vi "main ui.vi"() -> ()   [LabVIEW 2015]
uses:
  type def/basic params.ctl
  type def/advanced params.ctl
  type def/imaging mode.ctl
  type def/PXI control.ctl
  <instrlib>/niScope/Controls/niScope trigger source digital.ctl
  type def/NI tasks.ctl
  type def/do waveform.ctl
  type def/task plan.ctl
  type def/task status.ctl
  type def/motor panel.ctl
  type def/stage plan.ctl
  C:/Users/Administrator/Desktop/labview program/sub vi/XPS-UNIFIED/LabVIEW VIs/LabVIEW Source Code/Dll/Newport.XPS.CommandInterface.dll
  sub vi/XPS-UNIFIED/LabVIEW VIs/LabVIEW Source Code/Dll/Newport.XPS.CommandInterface.dll
  global variables/params.vi
  <instrlib>/niScope/Acquire/Fetch/niScope Multi Fetch Binary 16.vi
panel:
  in  "bi? for display":bool=TRUE
  in  "bi? for save":bool=TRUE
  out "t":dbl
  out "speed":dbl
  out "Y end":dbl
  out "main trigger":refnum<k21>
  out "XPS Ref":refnum<k24>
  out "PMT2 array size":i32[](array[numeric])
  out "PMT array size":i32[](array[numeric])
  in  "Stop stage":bool=TRUE
  out "stage state":string="exit"
  in  "stage plan":T1[][](array[typedef])
  in  "motor panel":T2={"X neg"=FALSE, "X pos"=FALSE, "dZ"=0.01, "X destination"=0.0, "Y destination"=0.0, "Z destination"=0.0, "Y pos"=FALSE, "Y neg"=FALSE, "Blank"=FALSE, "Blank 2"=FALSE, "X"=0.0, "Y"=0.0, "Z"=0.0, "X go"=FALSE, "Y go"=FALSE, "Z go"=FALSE, "Z pos"=FALSE, "Z neg"=FALSE, "dXY"=0.5} {"dXY" min=0.0 max=3.0 step=0.0001 format="%#.4f"; "Z" format="%#_6f"; "Y" format="%#_6f"; "X" format="%#_6f"; "Z destination" min=-13.0 max=10.0 step=0.001 format="%.3f"; "Y destination" min=-25.0 max=25.0 step=0.001 format="%.3f"; "X destination" min=-25.0 max=25.0 step=0.001 format="%.3f"; "dZ" min=0.0 max=1.0 step=0.0001 format="%#.4f"}
  out "do waveforms":T3[](array[typedef])
  out "images":i16[][][](array[numeric])
  out "NI tasks":T4
  in  "imaging mode":T5="continuous imaging"
  out "file path":path
  out "current state":string="exit"
  in  "Calc Waveform":bool
  in  "Stop":bool=TRUE
  in  "Acquire":bool
  in  "tab param":enum32{"basic", "advanced", "PXI", "task "}(tab)
  in  "basic params":T6={"X pixel #"=200, "X pixel size(um)"=1.0, "Y pixel #"=200, "Y pixel size(um)"=10.0, "line rate(Hz)"=1.0, "stage scan?"=FALSE} {"line rate(Hz)" min=1.0 max=2000.0 format="%#.3g"; "X pixel size(um)" min=0.0 max=10.0 format="%#.3g"; "X pixel #" min=2 max=20480 step=2 format="%#.3g"; "Y pixel size(um)" min=0.0 max=10.0 format="%#.3g"; "Y pixel #" min=2 max=204800 step=2 format="%#.3g"}
  in  "advanced params":T7={"x flyback time(%)"=40.0, "signal offset"=0, "frame time(s)"=0.0, "fetch # per frame"=1, "galvo sampling rate"=500000} {"galvo sampling rate" min=10000 max=200000 step=1; "fetch # per frame" min=1 max=1000 step=1 format="%#.3g"; "frame time(s)" min=0.0 max=100.0 step=0.1 format="%#.3g"; "signal offset" max=10000 format="%#.3g"; "x flyback time(%)" min=0.0 max=50.0 format="%#.3g"}
  in  "PXI channel":T8={"Vertical Range (V)"=1.0, "Min Sample Rate"=2208791.906743315, "# of Channels"=1, "Min Record Length"=560, "Number Of Records"=10000, "Trigger Position(%)"=0.0, "act Record Length"=1000, "trigger source"="VAL_EXTERNAL", "PMT2 # of Channels"=1} {"PMT2 # of Channels" min=1 max=8 step=1; "act Record Length" min=0 max=100000 step=1 format="%#.3g"; "Trigger Position(%)" min=0.0 max=100.0 format="%#.3p"; "Number Of Records" min=0 max=1000000 step=1 format="%#.3g"; "Min Record Length" min=0 max=10000 step=1; "# of Channels" min=1 max=8 step=1; "Min Sample Rate" min=0.0 max=100000000.0 format="%#.3p"; "Vertical Range (V)" min=0.0 max=10.0 format="%#.3g"}
  in  "task plan":T10={"X start"=0.0, "X end"=0.0, "X overlap"=0.0, "Y start"=20.0, "Y end"=0.0, "Z start"=0.0, "Z end"=0.0, "Z step size"=0.0, "start scan #"=0, "end scan #"=0} {"end scan #" min=1 step=1; "start scan #" min=1 step=1; "Z step size" min=-10.0 max=10.0 format="%#.6g"; "Z end" min=-12.0 max=12.0; "Z start" min=-12.0 max=12.0; "Y end" min=-20.0 max=20.0; "Y start" min=-20.0 max=20.0; "X overlap" min=0.0; "X end" min=-20.0 max=20.0; "X start" min=-20.0 max=20.0}
  in  "test plan":bool
  in  "save plan":bool
  in  "load plan":bool
  out "task status":T11
  in  "tab image":enum32{"Image", "Waveform"}(tab)
  in  "PMT channel":u8
  out "image":T12(plugin-control)
  out "current frame index":u16 caption="cn" format="%#.3g"
  in  "max":i32 format="%#.3g"
  in  "min":i32 format="%#.3g"
  in  "convesion":u32(ring)=15 items=["90% Dynamic"=15, "Given Range"=14]
  in  "acquisition finished":bool
  out "Enable error":i32
  out "waveform":dbl[](graph)
  in  "channel":cluster{"channel #":dbl, "signal":string}
  # "X"
  # "Y"
  # "Z"
  # "write"
  # "scan"
  # "in"
  # "z block"
  # "in"
  # "x block"
  # "in"
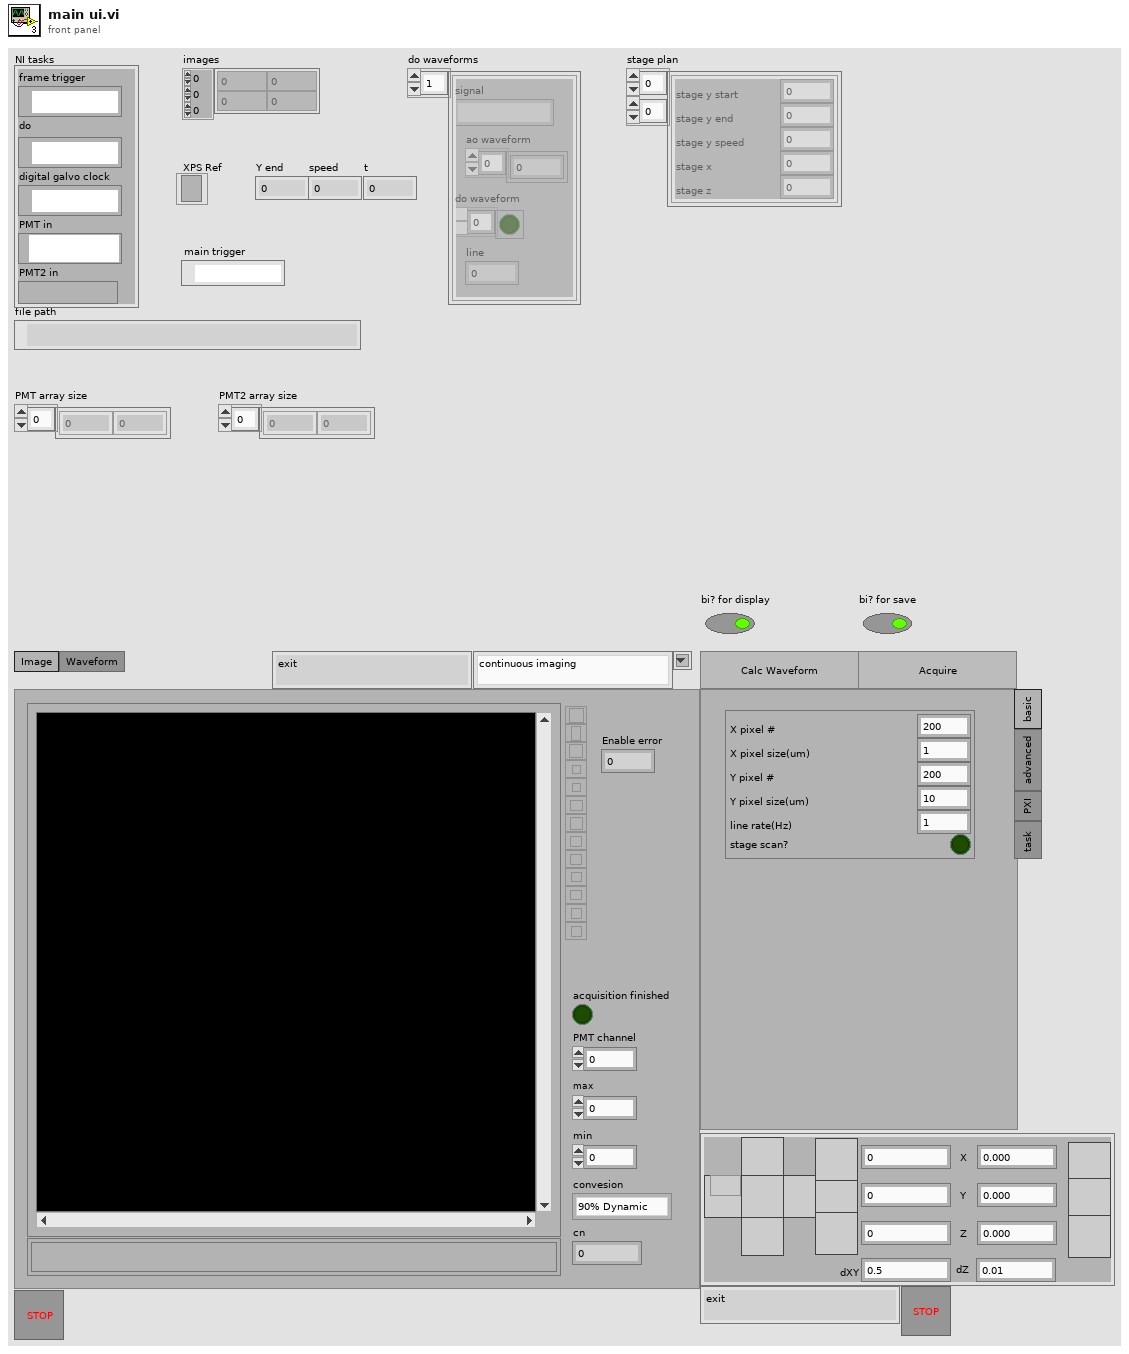
[diagram p1: front panel]
types:
  T1 = typedef "stage plan.ctl" = cluster{"stage y start":dbl, "stage y end":dbl, "stage y speed":dbl, "stage x":dbl, "stage z":dbl}
  T2 = typedef "motor panel.ctl" = cluster{"X neg":bool, "X pos":bool, "dZ":dbl, "X destination":dbl, "Y destination":dbl, "Z destination":dbl, "Y pos":bool, "Y neg":bool, "Blank":bool, "Blank 2":bool, "X":dbl, "Y":dbl, "Z":dbl, "X go":bool, "Y go":bool, "Z go":bool, "Z pos":bool, "Z neg":bool, "dXY":dbl}
  T3 = typedef "do waveform.ctl" = cluster{"signal":string, "ao waveform":dbl[], "do waveform":bool[], "line":u8}
  T4 = typedef "NI tasks.ctl" = cluster{"frame trigger":refnum<k21>, "do":refnum<k21>, "digital galvo clock":refnum<k21>, "PMT in":refnum<k15>, "PMT2 in":refnum<k15>}
  T5 = typedef "imaging mode.ctl" = string
  T6 = typedef "basic params.ctl" = cluster{"X pixel #":u32, "X pixel size(um)":dbl, "Y pixel #":u32, "Y pixel size(um)":dbl, "line rate(Hz)":dbl, "stage scan?":bool}
  T7 = typedef "advanced params.ctl" = cluster{"x flyback time(%)":dbl, "signal offset":u16, "frame time(s)":dbl, "fetch # per frame":u16, "galvo sampling rate":u32}
  T8 = typedef "PXI control.ctl" = cluster{"Vertical Range (V)":dbl, "Min Sample Rate":dbl, "# of Channels":u8, "Min Record Length":i32, "Number Of Records":i32, "Trigger Position(%)":dbl, "act Record Length":i32, "trigger source":T9, "PMT2 # of Channels":u8}
  T9 = typedef "niScope trigger source digital.ctl" = string
  T10 = typedef "task plan.ctl" = cluster{"X start":dbl, "X end":dbl, "X overlap":dbl, "Y start":dbl, "Y end":dbl, "Z start":dbl, "Z end":dbl, "Z step size":dbl, "start scan #":u16, "end scan #":u16}
  T11 = typedef "task status.ctl" = cluster{"xn":u16, "x total":u16, "zn":u16, "z total":u16, "scan n":u16, "scan total":u16, "write":u16}
  T12 = typedef "IMAQ Image.ctl" = refnum<image>
  T13 = enum8{"Enabled", "Disabled", "Disabled and Grayed Out"}
  T14 = typedef "Image Type" = u32
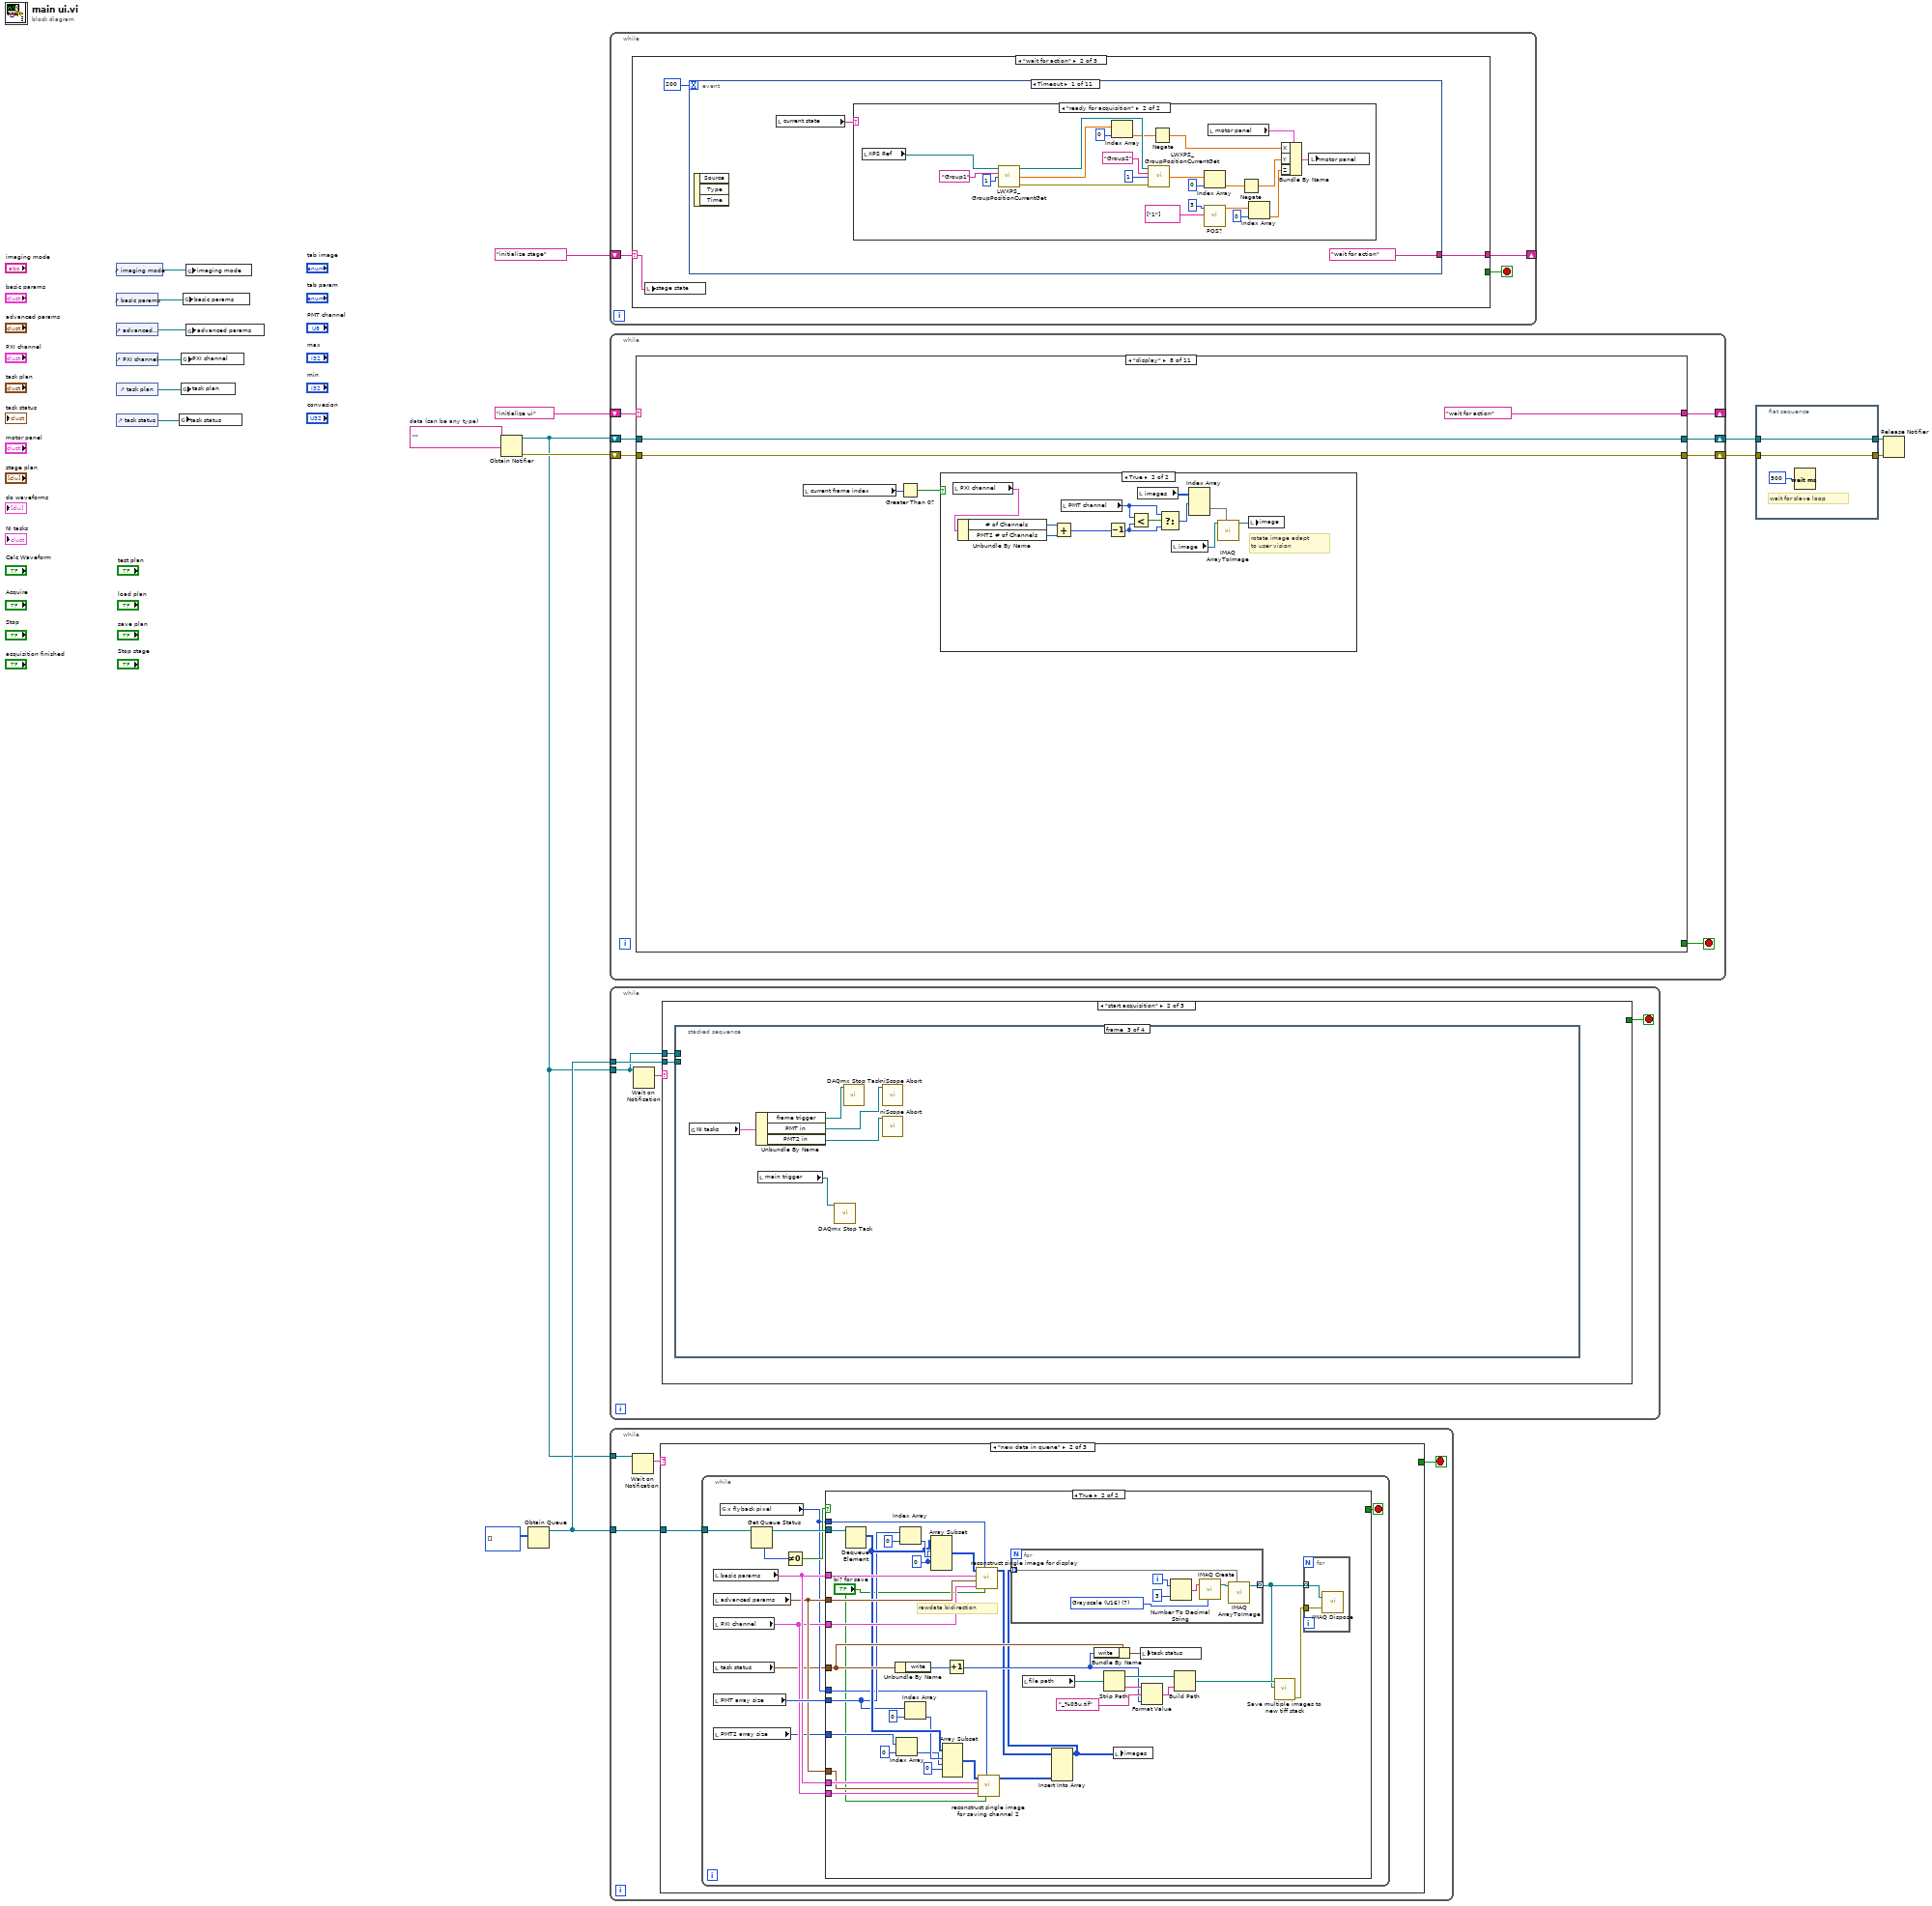
[diagram p0: block diagram]
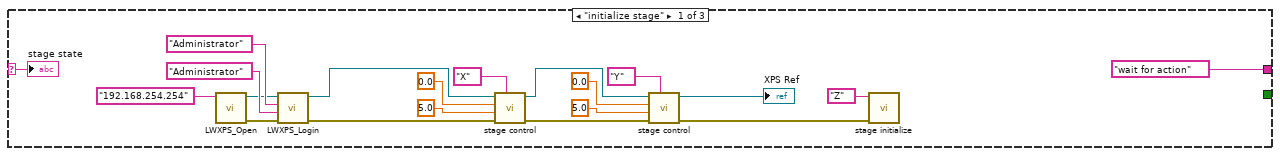
[diagram p2: hidden frame]
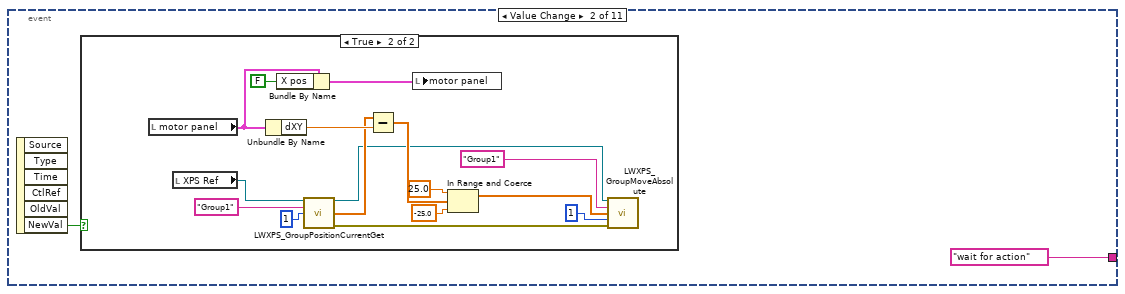
[diagram p4: hidden frame]
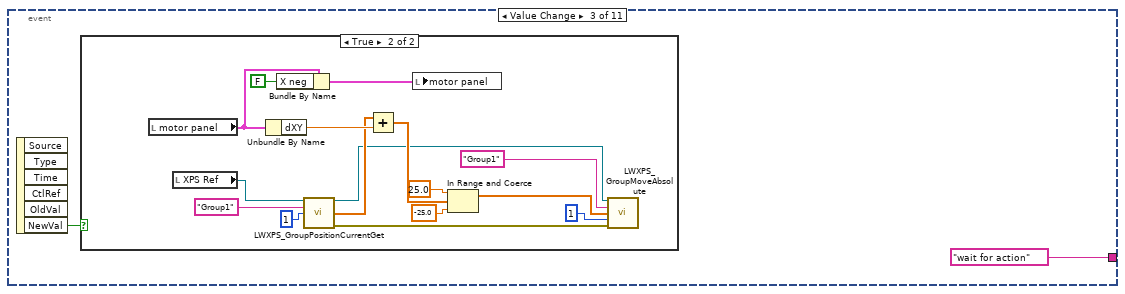
[diagram p6: hidden frame]
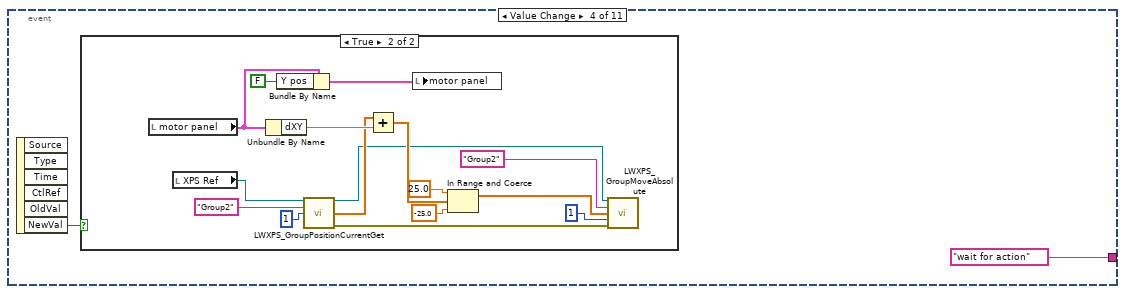
[diagram p8: hidden frame]
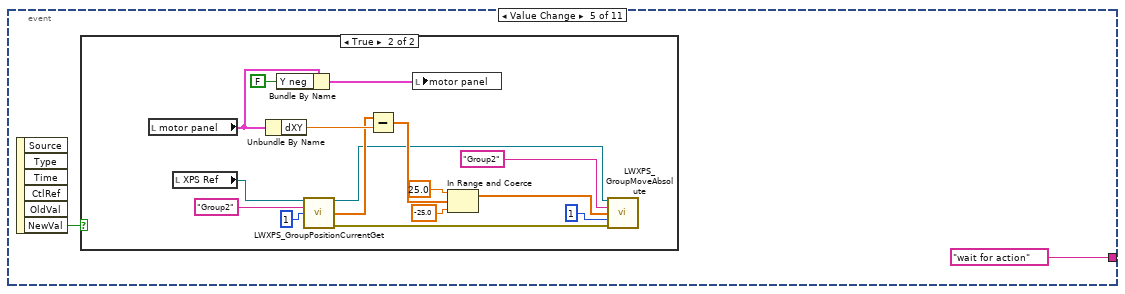
[diagram p10: hidden frame]
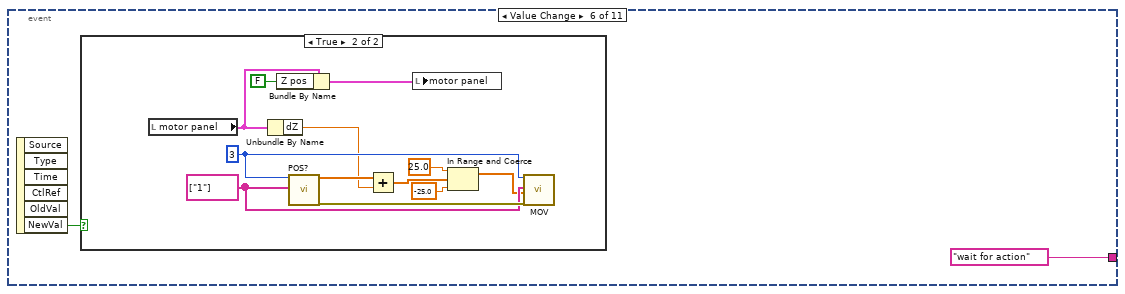
[diagram p12: hidden frame]
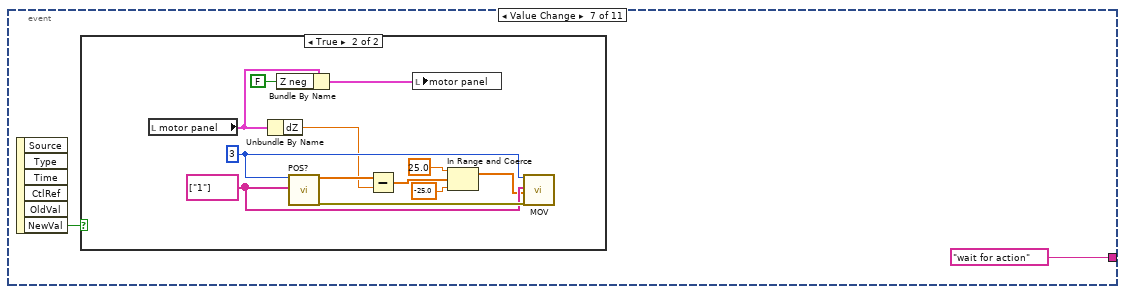
[diagram p14: hidden frame]
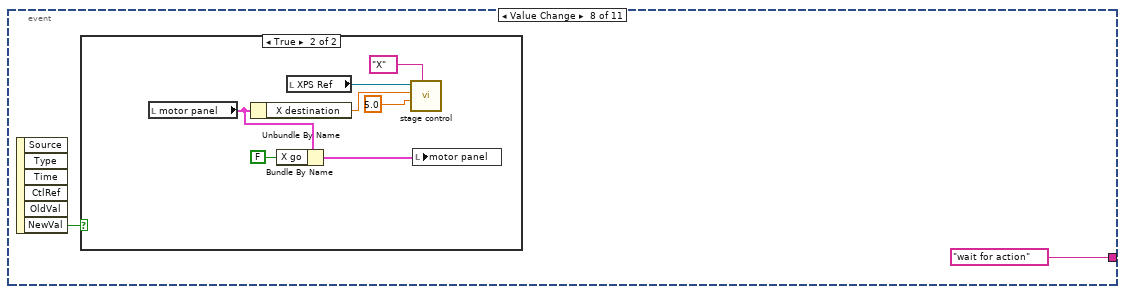
[diagram p16: hidden frame]
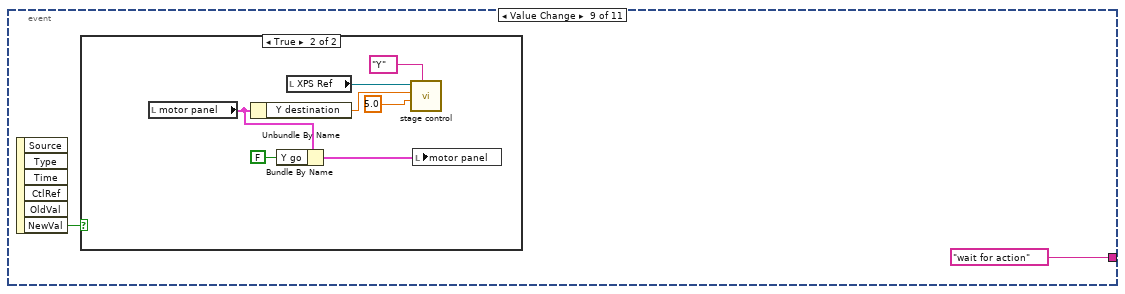
[diagram p18: hidden frame]
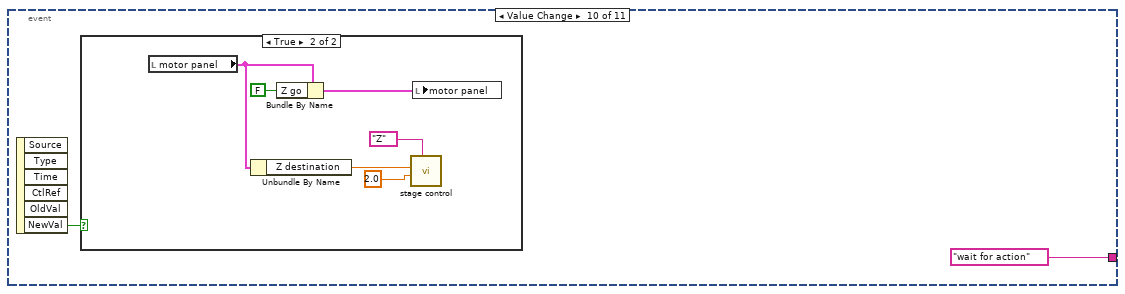
[diagram p20: hidden frame]
diagram:
  w16 = ""  # data (can be any type)
  n1 = control-ref of="imaging mode"() -> (w12:refnum<vi>)
  n2 = control-ref of="basic params"() -> (w14:refnum<vi>)
  n3 = control-ref of="advanced params"() -> (w13:refnum<vi>)
  n4 = control-ref of="PXI channel"() -> (w11:refnum<vi>)
  n5 = control-ref of="task plan"() -> (w4:refnum<vi>)
  n6 = control-ref of="task status"() -> (w2:refnum<vi>)
  n7 = global write "params.vi" "task status"(w2) -> ()
  n8 = global write "params.vi" "task plan"(w4) -> ()
  n9 = global write "params.vi" "PXI channel"(w11) -> ()
  n10 = global write "params.vi" "basic params"(w14) -> ()
  n11 = global write "params.vi" "imaging mode"(w12) -> ()
  n12 = global write "params.vi" "advanced params"(w13) -> ()
  n13 = Obtain Notifier(notification data type=w16) -> (notifier out=w3:refnum<notifier>, error out=w17:errorcluster)  [unwired: 2 in, 2 out]
  n14 = Obtain Queue(element data type=i16[][] []) -> (queue out=w10:refnum<queue>)  [unwired: 4 in, 2 out]
  n15 = while {
    shift-right: [w19] -> _
    shift-left: "initialize stage" -> [w20]
    stop <- w18 stop-if-true
    n16 = case shown="\"wait for action\"" w20 {
      selector: w20 -> [w40 w41 w200]
      tunnel: ["wait for action" w42 "exit"] -> w19
      tunnel: [_ _ TRUE] -> w18
      frame "initialize stage" {
        n17 = call "LWXPS_Open.vi"("Instrument Key IN"="192.168.254.254" ("address")) -> ("LabVIEW error OUT"=w35:errorcluster, "XPS Reference OUT"=w34:refnum<k24>)  [unwired: 3 in, 2 out]
        n18 = call "LWXPS_Login.vi"("LabVIEW error IN"=w35, "Password"="Administrator" ("User Name"), "User Name"="Administrator", "CommandInterfaceXPS.XPS"=w34) -> ("LabVIEW error OUT"=w32:errorcluster, "CommandInterfaceXPS.XPS"=w22:refnum<k24>)  [unwired: 2 in, 2 out]
        n19 = call "stage control.vi"("Combo Box"="X", "error in"=w32, "speed"=5.0, "target"=0.0, "XPS Ref in"=w22) -> ("error out"=w31:errorcluster, "XPS ref out"=w21:refnum<k24>)  [unwired: 5 in]
        n20 = call "stage control.vi"("Combo Box"="Y", "error in"=w31, "speed"=5.0, "target"=0.0, "XPS Ref in"=w21) -> ("error out"=w23:errorcluster, "XPS ref out"=→"XPS Ref":refnum<k24>)  [unwired: 5 in]
        n21 = call "stage initialize.vi"("error in"=w23, "Combo Box"="Z") -> ()  [unwired: 9 in, 1 out]
        "stage state" <- w40
      }
      frame "wait for action" {
        n22 = local write "stage state"(w41) -> ()
        n23 = event shown="[0] Timeout" {
          selector: _ -> [_ _ _ _ _ _ _ _ _ _ _]
          dyn-events: _ -> [_ _ _ _ _ _ _ _ _ _ _]
          timeout: 200 -> [_ _ _ _ _ _ _ _ _ _ _]
          tunnel: ["wait for action" "wait for action" "wait for action" "wait for action" "wait for action" "wait for action" "wait for action" "wait for action" "wait for action" "wait for action" "exit"] -> w42
          event Timeout {
            n24 = event-data() -> ()  [unwired: 1 in, 3 out]
            n25 = local read "current state"() -> (w44:string)
            n26 = case shown="\"ready for acquisition\"" w44 {
              frame "False", Default {
              }
              frame "ready for acquisition" {
                n27 = local read "XPS Ref"() -> (w47:refnum<k24>)
                n28 = call "LWXPS_GroupPositionCurrentGet.vi"("CommandInterfaceXPS.XPS"=w47, "Group Name"="Group1", "Number of positioners"=1) -> ("CommandInterfaceXPS.XPS"=w52:refnum<k24>, "Current Encoder Position"=w60:dbl[], "LabVIEW error OUT"=w46:errorcluster)  [unwired: 8 in, 2 out]
                n29 = Index Array(array=w60, index=0) -> (element=w51:dbl)
                n30 = call "LWXPS_GroupPositionCurrentGet.vi"("CommandInterfaceXPS.XPS"=w52, "Group Name"="Group2", "Number of positioners"=1, "LabVIEW error IN"=w46) -> ("Current Encoder Position"=w53:dbl[])  [unwired: 7 in, 4 out]
                n31 = Negate(x=w51) -> (-x=w50:dbl)
                n32 = Index Array(array=w53, index=0) -> (element=w48:dbl)
                n33 = call "POS?.vi"("System no."=3, "Axes to query"=string[] ["1"]) -> ("Position"=w59:dbl[])  [unwired: 3 in, 14 out]
                n34 = local read "motor panel"() -> (w67:T2)
                n35 = Negate(x=w48) -> (-x=w49:dbl)
                n36 = Index Array(array=w59, index=0) -> (element=w66:dbl)
                n37 = Bundle By Name(cluster=w67, "X"=w50, "Y"=w49, "Z"=w66) -> (w65:T2)
                n38 = local write "motor panel"(w65) -> ()
              }
            }
          }
          event Value Change {
            n39 = event-data() -> ("NewVal"=w69:bool)  [unwired: 1 in, 5 out]
            n40 = case shown="True" w69 {
              frame False {
              }
              frame True {
                n41 = local read "motor panel"() -> (w80:T2)
                n42 = local read "XPS Ref"() -> (w78:refnum<k24>)
                n43 = Unbundle By Name(w80) -> ("dXY"=w83:dbl)
                n44 = Bundle By Name(cluster=w80, "X pos"=FALSE) -> (w81:T2)
                n45 = call "LWXPS_GroupPositionCurrentGet.vi"("CommandInterfaceXPS.XPS"=w78, "Group Name"="Group1", "Number of positioners"=1) -> ("CommandInterfaceXPS.XPS"=w73:refnum<k24>, "Current Encoder Position"=w75:dbl[], "LabVIEW error OUT"=w72:errorcluster)  [unwired: 8 in, 2 out]
                n46 = Subtract(x=w75, y=w83) -> (x-y=w82:dbl[])
                n47 = local write "motor panel"(w81) -> ()
                n48 = In Range and Coerce(upper limit=25.0, x=w82, lower limit=-25.0) -> (coerced(x)=w74:dbl[])  [unwired: 1 out]
                n49 = call "LWXPS_GroupMoveAbsolute.vi"("CommandInterfaceXPS.XPS"=w73, "Group Name"="Group1", "Target Position IN"=w74, "Number of Positioners"=1, "LabVIEW error IN"=w72) -> ()  [unwired: 6 in, 5 out]
              }
            }
          }
          event Value Change {
            n50 = event-data() -> ("NewVal"=w87:bool)  [unwired: 1 in, 5 out]
            n51 = case shown="True" w87 {
              frame False {
              }
              frame True {
                n52 = local read "motor panel"() -> (w98:T2)
                n53 = local read "XPS Ref"() -> (w96:refnum<k24>)
                n54 = Unbundle By Name(w98) -> ("dXY"=w101:dbl)
                n55 = Bundle By Name(cluster=w98, "X neg"=FALSE ("X pos")) -> (w99:T2)
                n56 = call "LWXPS_GroupPositionCurrentGet.vi"("CommandInterfaceXPS.XPS"=w96, "Group Name"="Group1", "Number of positioners"=1) -> ("CommandInterfaceXPS.XPS"=w91:refnum<k24>, "Current Encoder Position"=w93:dbl[], "LabVIEW error OUT"=w90:errorcluster)  [unwired: 8 in, 2 out]
                n57 = Add(x=w93, y=w101) -> (x+y=w100:dbl[])
                n58 = local write "motor panel"(w99) -> ()
                n59 = In Range and Coerce(upper limit=25.0, x=w100, lower limit=-25.0) -> (coerced(x)=w92:dbl[])  [unwired: 1 out]
                n60 = call "LWXPS_GroupMoveAbsolute.vi"("CommandInterfaceXPS.XPS"=w91, "Group Name"="Group1", "Target Position IN"=w92, "Number of Positioners"=1, "LabVIEW error IN"=w90) -> ()  [unwired: 6 in, 5 out]
              }
            }
          }
          event Value Change {
            n61 = event-data() -> ("NewVal"=w105:bool)  [unwired: 1 in, 5 out]
            n62 = case shown="True" w105 {
              frame False {
              }
              frame True {
                n63 = local read "motor panel"() -> (w116:T2)
                n64 = local read "XPS Ref"() -> (w114:refnum<k24>)
                n65 = Unbundle By Name(w116) -> ("dXY"=w119:dbl)
                n66 = Bundle By Name(cluster=w116, "Y pos"=FALSE ("X pos")) -> (w117:T2)
                n67 = call "LWXPS_GroupPositionCurrentGet.vi"("CommandInterfaceXPS.XPS"=w114, "Group Name"="Group2", "Number of positioners"=1) -> ("CommandInterfaceXPS.XPS"=w109:refnum<k24>, "Current Encoder Position"=w111:dbl[], "LabVIEW error OUT"=w108:errorcluster)  [unwired: 8 in, 2 out]
                n68 = Add(x=w111, y=w119) -> (x+y=w118:dbl[])
                n69 = local write "motor panel"(w117) -> ()
                n70 = In Range and Coerce(upper limit=25.0, x=w118, lower limit=-25.0) -> (coerced(x)=w110:dbl[])  [unwired: 1 out]
                n71 = call "LWXPS_GroupMoveAbsolute.vi"("CommandInterfaceXPS.XPS"=w109, "Group Name"="Group2", "Target Position IN"=w110, "Number of Positioners"=1, "LabVIEW error IN"=w108) -> ()  [unwired: 6 in, 5 out]
              }
            }
          }
          event Value Change {
            n72 = event-data() -> ("NewVal"=w123:bool)  [unwired: 1 in, 5 out]
            n73 = case shown="True" w123 {
              frame False {
              }
              frame True {
                n74 = local read "motor panel"() -> (w134:T2)
                n75 = local read "XPS Ref"() -> (w132:refnum<k24>)
                n76 = Unbundle By Name(w134) -> ("dXY"=w137:dbl)
                n77 = Bundle By Name(cluster=w134, "Y neg"=FALSE ("X pos")) -> (w135:T2)
                n78 = call "LWXPS_GroupPositionCurrentGet.vi"("CommandInterfaceXPS.XPS"=w132, "Group Name"="Group2", "Number of positioners"=1) -> ("CommandInterfaceXPS.XPS"=w127:refnum<k24>, "Current Encoder Position"=w129:dbl[], "LabVIEW error OUT"=w126:errorcluster)  [unwired: 8 in, 2 out]
                n79 = Subtract(x=w129, y=w137) -> (x-y=w136:dbl[])
                n80 = local write "motor panel"(w135) -> ()
                n81 = In Range and Coerce(upper limit=25.0, x=w136, lower limit=-25.0) -> (coerced(x)=w128:dbl[])  [unwired: 1 out]
                n82 = call "LWXPS_GroupMoveAbsolute.vi"("CommandInterfaceXPS.XPS"=w127, "Group Name"="Group2", "Target Position IN"=w128, "Number of Positioners"=1, "LabVIEW error IN"=w126) -> ()  [unwired: 6 in, 5 out]
              }
            }
          }
          event Value Change {
            n83 = event-data() -> ("NewVal"=w140:bool)  [unwired: 1 in, 5 out]
            n84 = case shown="True" w140 {
              frame False {
              }
              frame True {
                w149 = 3 ("System no.")
                w150 = string[] ["1"] ("Axes to query")
                n85 = local read "motor panel"() -> (w143:T2)
                n86 = Unbundle By Name(w143) -> ("dZ"=w147:dbl)
                n87 = Bundle By Name(cluster=w143, "Z pos"=FALSE ("X pos")) -> (w144:T2)
                n88 = call "POS?.vi"("System no."=w149, "Axes to query"=w150) -> ("Position"=w148:dbl[], "error out"=w153:errorcluster)  [unwired: 3 in, 13 out]
                n89 = Add(x=w148, y=w147) -> (x+y=w146:dbl[])
                n90 = local write "motor panel"(w144) -> ()
                n91 = In Range and Coerce(upper limit=25.0, x=w146, lower limit=-25.0) -> (coerced(x)=w145:dbl[])  [unwired: 1 out]
                n92 = call "MOV.vi"("System no."=w149, "Axes to move"=w150, "Position values"=w145, "error in"=w153) -> ()  [unwired: 1 in, 15 out]
              }
            }
          }
          event Value Change {
            n93 = event-data() -> ("NewVal"=w154:bool)  [unwired: 1 in, 5 out]
            n94 = case shown="True" w154 {
              frame False {
              }
              frame True {
                w163 = 3 ("System no.")
                w164 = string[] ["1"] ("Axes to query")
                n95 = local read "motor panel"() -> (w157:T2)
                n96 = Unbundle By Name(w157) -> ("dZ"=w161:dbl)
                n97 = Bundle By Name(cluster=w157, "Z neg"=FALSE ("X pos")) -> (w158:T2)
                n98 = call "POS?.vi"("System no."=w163, "Axes to query"=w164) -> ("Position"=w162:dbl[], "error out"=w167:errorcluster)  [unwired: 3 in, 13 out]
                n99 = Subtract(x=w162, y=w161) -> (x-y=w160:dbl[])
                n100 = local write "motor panel"(w158) -> ()
                n101 = In Range and Coerce(upper limit=25.0, x=w160, lower limit=-25.0) -> (coerced(x)=w159:dbl[])  [unwired: 1 out]
                n102 = call "MOV.vi"("System no."=w163, "Axes to move"=w164, "Position values"=w159, "error in"=w167) -> ()  [unwired: 1 in, 15 out]
              }
            }
          }
          event Value Change {
            n103 = event-data() -> ("NewVal"=w168:bool)  [unwired: 1 in, 5 out]
            n104 = case shown="True" w168 {
              frame False {
              }
              frame True {
                n105 = local read "motor panel"() -> (w175:T2)
                n106 = Unbundle By Name(w175) -> ("X destination"=w170:dbl)
                n107 = Bundle By Name(cluster=w175, "X go"=FALSE ("X pos")) -> (w176:T2)
                n108 = local read "XPS Ref"() -> (w173:refnum<k24>)
                n109 = call "stage control.vi"("Combo Box"="X", "speed"=5.0, "target"=w170, "XPS Ref in"=w173) -> ()  [unwired: 6 in, 2 out]
                n110 = local write "motor panel"(w176) -> ()
              }
            }
          }
          event Value Change {
            n111 = event-data() -> ("NewVal"=w178:bool)  [unwired: 1 in, 5 out]
            n112 = case shown="True" w178 {
              frame False {
              }
              frame True {
                n113 = local read "motor panel"() -> (w184:T2)
                n114 = Unbundle By Name(w184) -> ("Y destination"=w179:dbl)
                n115 = Bundle By Name(cluster=w184, "Y go"=FALSE ("X pos")) -> (w185:T2)
                n116 = local read "XPS Ref"() -> (w182:refnum<k24>)
                n117 = call "stage control.vi"("Combo Box"="Y", "speed"=5.0, "target"=w179, "XPS Ref in"=w182) -> ()  [unwired: 6 in, 2 out]
                n118 = local write "motor panel"(w185) -> ()
              }
            }
          }
          event Value Change {
            n119 = event-data() -> ("NewVal"=w187:bool)  [unwired: 1 in, 5 out]
            n120 = case shown="True" w187 {
              frame False {
              }
              frame True {
                n121 = local read "motor panel"() -> (w191:T2)
                n122 = Unbundle By Name(w191) -> ("Z destination"=w188:dbl)
                n123 = Bundle By Name(cluster=w191, "Z go"=FALSE ("X pos")) -> (w193:T2)
                n124 = call "stage control.vi"("Combo Box"="Z", "speed"=2.0, "target"=w188) -> ()  [unwired: 7 in, 2 out]
                n125 = local write "motor panel"(w193) -> ()
              }
            }
          }
          event "Stop stage": Value Change {
            n126 = event-data() -> ()  [unwired: 1 in, 6 out]
          }
        }
      }
      frame "exit", Default {
        w197 = 3 ("System no.")
        n127 = local write "stage state"(w200) -> ()
        n128 = call "SVO.vi"("System no."=w197, "Axes to command"=string[] ["1"], "Servo mode"=bool[] [FALSE]) -> ("error out"=w198:errorcluster)  [unwired: 2 in, 14 out]
        n129 = call "Close connection if open.vi"("System no."=w197, "error in"=w198) -> ()  [unwired: 1 in, 17 out]
      }
    }
  }
  n130 = while {
    shift-right: [w205] -> w5
    shift-left: w17 -> [w206]
    shift-right: [w207] -> w9
    shift-left: w3 -> [w208]
    shift-right: [w202] -> _
    shift-left: "initialize ui" -> [w203]
    stop <- w204 stop-if-true
    n131 = case shown="\"display\"" w203 {
      selector: w203 -> [w220 w230 _ w301 w328 w374 w421 _ w444 w533 w552]
      tunnel: w208 -> [w226 w228 w232 w302 w321 w369 w420 w426 w442 w535 w550]
      tunnel: [w226 w228 w232 w302 w321 w373 w420 w426 w442 w535 w549] -> w207
      tunnel: w206 -> [w211 w227 w231 w300 w319 w371 w419 w425 w441 w534 w548]
      tunnel: [w211 w227 w231 w300 w319 w367 w419 w425 w441 w534 w547] -> w205
      tunnel: [_ _ _ _ _ _ _ _ _ _ TRUE] -> w204
      tunnel: ["ready for acquisition" "wait for action" w233 "ready for acquisition" "start acquisition" "during acquisition" "wait for action" "wait for action" w443 "ready for acquisition" "exit"] -> w202
      frame "initialize ui" {
        w212 = u32 15 items=["Default"=10, "Most Significant Bits"=11, "Full Dynamic"=12, "Downshift"=13, "Given Range"=14, "90% Dynamic"=15, "Given Percent Range"=16] ("16-bit Display Mapping:Conversion Method")
        w218 = u32 0 items=["90% Dynamic", "Given Range"] ("convesion")
        w223 = T14 7 items=["Grayscale (U8)", "Grayscale (I16)", "Grayscale (SGL)", "Complex (CSG)", "RGB (U32)", "HSL (U32)", "RGB (U64)", "Grayscale (U16)"] ("Image Type")
        w214 = T13."Enabled" ("Disabled")
        w215 = FALSE ("Stop")
        # "1. load system configuration\n2. load last configuration\n3. initialize image window\n4. initialize all buttons"
        n132 = call "load system configuration.vi"() -> ("error out"=w224:errorcluster)  [unwired: 11 in]
        n133 = local write "min"(0 ("min")) -> ()
        n134 = call <vilib>:"Application Directory.vi"() -> ("Application Directory"=w210:path)
        n135 = local write "max"(1000 ("max")) -> ()
        n136 = call "load last configuration.vi"("error in (no error)"=w224, "name or relative path"="last configuration.ini", "base path"=w210) -> ()  [unwired: 8 in, 1 out]
        n137 = local write "convesion"(w218) -> ()
        n138 = property on="image" class="ImageControl"("16-bit Display Conversion Method"=w212) -> ()  [unwired: 2 in, 2 out]
        n139 = call "IMAQ Create"("Image Name"="image", "Image Type"=w223) -> ("New Image"=→"image":T12)  [unwired: 3 in, 1 out]
        n140 = local write "Acquire"(w215) -> ()
        n141 = local write "Calc Waveform"(w215) -> ()
        n142 = local write "Stop"(w215) -> ()
        n143 = local write "acquisition finished"(w215) -> ()
        n144 = local write "load plan"(w215) -> ()
        n145 = local write "test plan"(w215) -> ()
        n146 = local write "save plan"(w215) -> ()
        n147 = local write "Stop stage"(w215) -> ()
        n148 = property on="Acquire" class="Bool (strict)"("DisabledEnum"=T13."Disabled and Grayed Out" ("Disabled")) -> ()  [unwired: 2 in, 2 out]
        n149 = property on="Calc Waveform" class="Bool (strict)"("DisabledEnum"=w214) -> ()  [unwired: 2 in, 2 out]
        n150 = property on="imaging mode" class="CmbBox (strict)"("DisabledEnum"=w214) -> ()  [unwired: 2 in, 2 out]
        n151 = property on="Stop stage" class="Bool (strict)"("DisabledEnum"=w214) -> ()  [unwired: 2 in, 2 out]
        n152 = property on="advanced params" class="Clust (strict)"("DisabledEnum"=w214) -> ()  [unwired: 2 in, 2 out]
        n153 = property on="motor panel" class="Clust (strict)"("DisabledEnum"=w214) -> ()  [unwired: 2 in, 2 out]
        n154 = property on="PXI channel" class="Clust (strict)"("DisabledEnum"=w214) -> ()  [unwired: 2 in, 2 out]
        n155 = property on="Stop" class="Bool (strict)"("DisabledEnum"=w214) -> ()  [unwired: 2 in, 2 out]
        n156 = property on="task plan" class="Clust (strict)"("DisabledEnum"=w214) -> ()  [unwired: 2 in, 2 out]
        n157 = property on="basic params" class="Clust (strict)"("DisabledEnum"=w214) -> ()  [unwired: 2 in, 2 out]
        "current state" <- w220
        "current frame index" <- u16 0 ("current frame index")
      }
      frame "ready for acquisition" {
        n158 = local write "current state"(w230) -> ()
      }
      frame "wait for action" {
        n159 = event shown="[0] Timeout" {
          selector: _ -> [_ _ _ _ _ _ _ _ _ _]
          dyn-events: _ -> [_ _ _ _ _ _ _ _ _ _]
          timeout: 100 -> [_ _ _ _ _ _ _ _ _ _]
          tunnel: [w236 "wait for action" "wait for action" "wait for action" w263 w269 w282 w288 w294 "exit"] -> w233
          event Timeout {
            n160 = event-data() -> ()  [unwired: 1 in, 3 out]
            n161 = local read "current state"() -> (w235:string)
            n162 = case shown="\"during acquisition\"" w235 {
              tunnel: ["wait for action" w239] -> w236
              frame "False", Default {
              }
              frame "during acquisition" {
                # "acquisition is running?"
                n163 = local read "acquisition finished"() -> (w238:bool)
                n164 = case shown="False" w238 {
                  tunnel: ["display" "finish acquisition"] -> w239
                  frame False {
                    # "acquiring"
                  }
                  frame True {
                  }
                }
              }
            }
          }
          event "load plan": Value Change {
            n165 = event-data() -> ("NewVal"=w242:bool)  [unwired: 1 in]
            n166 = case shown="True" w242 {
              frame False {
              }
              frame True {
                n167 = call "File Dialog"() -> ("selected path"=w246:path, "exists"=w244:bool, "cancelled"=w245:bool)  [unwired: 12 in, 1 out]
                n168 = property on="load plan" class="Bool (strict)"("Value"=FALSE) -> ()  [unwired: 2 in, 2 out]
                n169 = case shown="False" w245 {
                  tunnel: w246 -> [w249 _]
                  tunnel: w244 -> [w248 _]
                  frame False {
                    n170 = case shown="True" w248 {
                      tunnel: w249 -> [_ w251]
                      frame False {
                      }
                      frame True {
                        n171 = call "load last configuration.vi"("name or relative path"="", "base path"=w251) -> ()  [unwired: 9 in, 1 out]
                      }
                    }
                  }
                  frame True {
                  }
                }
              }
            }
          }
          event "save plan": Value Change {
            n172 = event-data() -> ("NewVal"=w253:bool)  [unwired: 1 in]
            n173 = case shown="True" w253 {
              frame False {
              }
              frame True {
                n174 = property on="save plan" class="Bool (strict)"("Value"=FALSE) -> ()  [unwired: 2 in, 2 out]
                n175 = call "File Dialog3"() -> ("selected path"=w255:path, "cancelled"=w254:bool)  [unwired: 12 in, 2 out]
                n176 = case shown="False" w254 {
                  tunnel: w255 -> [w258 _]
                  frame False {
                    n177 = call "save configuration.vi"("filename"="", "path"=w258) -> ()  [unwired: 9 in, 1 out]
                  }
                  frame True {
                  }
                }
              }
            }
          }
          event "test plan": Value Change {
            n178 = event-data() -> ("NewVal"=w259:bool)  [unwired: 1 in]
            n179 = case shown="True" w259 {
              frame False {
              }
              frame True {
                n180 = flat-sequence {
                  frame #0 {
                    n181 = call "calc waveforms.vi"() -> ()  [unwired: 10 in, 1 out]
                  }
                  frame #1 {
                    n182 = call "generate task plan.vi"() -> ()  [unwired: 10 in, 2 out]
                  }
                  frame #2 {
                    n183 = property on="test plan" class="Bool (strict)"("Value"=FALSE) -> ()  [unwired: 2 in, 2 out]
                  }
                }
                n184 = Wait (ms)(milliseconds to wait=u32 100) -> ()  [unwired: 1 out]
              }
            }
          }
          event "Calc Waveform": Value Change {
            n185 = event-data() -> ("NewVal"=w264:bool)  [unwired: 1 in]
            n186 = case shown="True" w264 {
              tunnel: ["wait for action" "calculate waveforms"] -> w263
              frame False {
              }
              frame True {
              }
            }
          }
          event "Acquire": Value Change {
            n187 = event-data() -> ("NewVal"=w268:bool)  [unwired: 1 in]
            n188 = local read "current state"() -> (w267:string)
            n189 = case shown="\"during acquisition\"" w267 {
              tunnel: ["wait for action" w272 w276] -> w269
              tunnel: w268 -> [_ w271 w275]
              frame "False", Default {
              }
              frame "ready for acquisition" {
                n190 = case shown="False" w271 {
                  tunnel: ["wait for action" "start task"] -> w272
                  frame False {
                  }
                  frame True {
                    # "aquire"
                  }
                }
              }
              frame "during acquisition" {
                n191 = case shown="False" w275 {
                  tunnel: ["finish task" "wait for action"] -> w276
                  frame False {
                    # "abort"
                    n192 = while {
                      stop <- w279 stop-if-true
                      n193 = Wait (ms)(milliseconds to wait=u32 100) -> ()  [unwired: 1 out]
                      n194 = local read "acquisition finished"() -> (w279:bool)
                    }
                  }
                  frame True {
                  }
                }
              }
            }
          }
          event "max": Value Change {
            n195 = event-data() -> ("NewVal"=w283:i32)  [unwired: 1 in]
            n196 = local read "current state"() -> (w281:string)
            n197 = case shown="\"during acquisition\", \"ready for acquisition\"" w281 {
              tunnel: w283 -> [_ w285]
              tunnel: ["wait for action" "wait for action"] -> w282
              frame "False", Default {
              }
              frame "during acquisition", "ready for acquisition" {
                n198 = property on="image" class="ImageControl"("16-bit Display Maximum Value"=w285) -> ()  [unwired: 2 in, 2 out]
              }
            }
          }
          event "min": Value Change {
            n199 = event-data() -> ("NewVal"=w289:i32)  [unwired: 1 in]
            n200 = local read "current state"() -> (w287:string)
            n201 = case shown="\"during acquisition\", \"ready for acquisition\"" w287 {
              tunnel: w289 -> [_ w291]
              tunnel: ["wait for action" "wait for action"] -> w288
              frame "False", Default {
              }
              frame "during acquisition", "ready for acquisition" {
                n202 = property on="image" class="ImageControl"("16-bit Display Minimum Value"=w291) -> ()  [unwired: 2 in, 2 out]
              }
            }
          }
          event "convesion": Value Change {
            n203 = event-data() -> ("NewVal"=w295:u32)  [unwired: 1 in]
            n204 = local read "current state"() -> (w293:string)
            n205 = case shown="\"during acquisition\", \"ready for acquisition\"" w293 {
              tunnel: w295 -> [_ w297]
              tunnel: ["wait for action" "wait for action"] -> w294
              frame "False", Default {
              }
              frame "during acquisition", "ready for acquisition" {
                n206 = property on="image" class="ImageControl"("16-bit Display Conversion Method"=w297) -> ()  [unwired: 2 in, 2 out]
              }
            }
          }
          event "Stop": Value Change {
            n207 = event-data() -> ()  [unwired: 1 in, 1 out]
          }
        }
      }
      frame "calculate waveforms" {
        n208 = local write "current state"(w301) -> ()
        n209 = flat-sequence {
          frame #0 {
            n210 = call "calc waveforms.vi"() -> ("do waveforms"=w304:T3[])  [unwired: 10 in]
            n211 = Unbundle By Name("channel") -> ("channel #"=w309:dbl)
            n212 = Index Array(array=w304, index=w309) -> (element=w307:T3)
            n213 = local write "do waveforms"(w304) -> ()
            n214 = Unbundle By Name(w307) -> ("ao waveform"=→"waveform":dbl[], "signal"=w305:string)
            n215 = Bundle By Name(cluster="channel", "signal"=w305) -> (w310:cluster{"channel #":dbl, "signal":string})
            n216 = local write "channel"(w310) -> ()
          }
          frame #1 {
            n217 = local read "motor panel"() -> (w315:T2)
            n218 = Unbundle By Name(w315) -> ("Y destination"=w314:dbl)
            n219 = local read "basic params"() -> (w316:T6)
            n220 = call "calc parameters.vi"("Y start"=w314, "basic params"=w316) -> ("t"=→"t":dbl, "speed"=→"speed":dbl, "Y end"=→"Y end":dbl)  [unwired: 7 in]
          }
          frame #2 {
            n221 = property on="Calc Waveform" class="Bool (strict)"("Value"=FALSE ("Calc Waveform")) -> ()  [unwired: 2 in, 2 out]
            n222 = property on="Acquire" class="Bool (strict)"("DisabledEnum"=T13."Enabled" ("Disabled")) -> ()  [unwired: 2 in, 2 out]
          }
        }
      }
      frame "start task" {
        w323 = T13."Disabled and Grayed Out" ("Disabled")
        n223 = local write "current state"(w328) -> ()
        n224 = local write "current frame index"(u16 0 ("current frame index")) -> ()
        n225 = local write "acquisition finished"(FALSE ("acquisition finished")) -> ()
        n226 = local read "imaging mode"() -> (w326:T5)
        n227 = property on="imaging mode" class="CmbBox (strict)"("DisabledEnum"=w323) -> ()  [unwired: 2 in, 2 out]
        n228 = property on="Calc Waveform" class="Bool (strict)"("DisabledEnum"=w323) -> ()  [unwired: 2 in, 2 out]
        n229 = property on="advanced params" class="Clust (strict)"("DisabledEnum"=w323) -> ()  [unwired: 2 in, 2 out]
        n230 = property on="Stop" class="Bool (strict)"("DisabledEnum"=w323) -> ()  [unwired: 2 in, 2 out]
        n231 = property on="basic params" class="Clust (strict)"("DisabledEnum"=w323) -> ()  [unwired: 2 in, 2 out]
        n232 = property on="PXI channel" class="Clust (strict)"("DisabledEnum"=w323) -> ()  [unwired: 2 in, 2 out]
        n233 = property on="task plan" class="Clust (strict)"("DisabledEnum"=w323) -> ()  [unwired: 2 in, 2 out]
        n234 = case shown="\"task imaging\"" w326 {
          tunnel: [w329 w339] -> w322
          frame "preview imaging", Default {
            n235 = stacked-sequence {
              tunnel: [w330 _] -> w329
              frame #0 {
                n236 = call "digital galvo position ver2.vi"() -> ()  [unwired: 11 in, 1 out]
                n237 = local read "do waveforms"() -> (w330:T3[])
              }
              frame #1 {
                n238 = local read "basic params"() -> (w332:T6)
                n239 = Unbundle By Name(w332) -> ("stage scan?"=w331:bool)
                n240 = case shown="True" w331 {
                  frame False {
                  }
                  frame True {
                    n241 = local read "XPS Ref"() -> (w337:refnum<k24>)
                    n242 = local read "motor panel"() -> (w334:T2)
                    n243 = Wait (ms)(milliseconds to wait=u32 500) -> ()  [unwired: 1 out]
                    n244 = Unbundle By Name(w334) -> ("Y destination"=w333:dbl)
                    n245 = call "stage control.vi"("Combo Box"="Y", "speed"=10.0, "target"=w333, "XPS Ref in"=w337) -> ()  [unwired: 6 in, 2 out]
                  }
                }
              }
            }
          }
          frame "task imaging" {
            n246 = stacked-sequence {
              tunnel: [w343 _] -> w339
              frame #0 {
                n247 = call "File Dialog2"() -> ("selected path"=w342:path, "cancelled"=w341:bool)  [unwired: 12 in, 2 out]
                n248 = property on="motor panel" class="Clust (strict)"("DisabledEnum"=T13."Disabled and Grayed Out" ("Disabled")) -> ()  [unwired: 2 in, 2 out]
                n249 = case shown="False" w341 {
                  tunnel: w342 -> [w345 _]
                  frame False {
                    "file path" <- w345
                  }
                  frame True {
                  }
                }
                n250 = call "digital galvo position ver2.vi"() -> ()  [unwired: 11 in, 1 out]
                n251 = call "generate task plan.vi"() -> ("stage plan"=w344:T1[][], "do waveforms"=w343:T3[])  [unwired: 10 in]
                n252 = local write "stage plan"(w344) -> ()
                n253 = local write "do waveforms"(w343) -> ()
              }
              frame #1 {
                w361 = 10.0 ("stage y start")
                # "reset position"
                n254 = local read "task status"() -> (w365:T11)
                n255 = Wait (ms)(milliseconds to wait=u32 10000) -> ()  [unwired: 1 out]
                n256 = Unbundle By Name(w365) -> ("zn"=w364:u16, "xn"=w363:u16)
                n257 = local read "stage plan"() -> (w366:T1[][])
                n258 = Decrement(x=w364) -> (x-1=w358:u16)
                n259 = Decrement(x=w363) -> (x-1=w357:u16)
                n260 = Index Array(array=w366, index (row)=w358, index (col)=w357) -> (element=w362:T1)
                n261 = Unbundle By Name(w362) -> ("stage x"=w354:dbl, "stage y start"=w346:dbl, "stage z"=w353:dbl)
                n262 = local read "XPS Ref"() -> (w349:refnum<k24>)
                n263 = call "stage control.vi"("Combo Box"="X", "speed"=w361, "target"=w354, "XPS Ref in"=w349) -> ("error out"=w359:errorcluster, "XPS ref out"=w348:refnum<k24>)  [unwired: 6 in]
                n264 = call "stage control.vi"("Combo Box"="Y", "error in"=w359, "speed"=w361, "target"=w346, "XPS Ref in"=w348) -> ("error out"=w356:errorcluster, "XPS ref out"=w347:refnum<k24>)  [unwired: 5 in]
                n265 = call "stage control.vi"("Combo Box"="Z", "error in"=w356, "speed"=5.0 ("stage y start"), "target"=w353, "XPS Ref in"=w347) -> ()  [unwired: 5 in, 2 out]
              }
            }
          }
        }
        n266 = call "initialize NI card.vi"("do waveforms"=w322) -> ("main trigger"=→"main trigger":refnum<k21>)  [unwired: 13 in, 1 out]
      }
      frame "start acquisition" {
        n267 = local write "current state"(w374) -> ()
        n268 = local read "imaging mode"() -> (w368:T5)
        n269 = case shown="\"task imaging\"" w368 {
          frame "preview imaging", Default {
            n270 = local read "basic params"() -> (w376:T6)
            n271 = Unbundle By Name(w376) -> ("stage scan?"=w377:bool)
            n272 = case shown="True" w377 {
              frame False {
              }
              frame True {
                n273 = stacked-sequence {
                  frame #0 {
                    n274 = global read "params.vi" "NI tasks"() -> (w381:T4)
                    n275 = Unbundle By Name(w381) -> ("frame trigger"=w383:refnum<k21>, "do"=w379:refnum<k21>, "digital galvo clock"=w382:refnum<k21>)
                    n276 = call <vilib>:"DAQmx Start Task.vi"("task/channels in"=w382) -> ("error out"=w378:errorcluster)  [unwired: 13 in, 1 out]
                    n277 = local read "main trigger"() -> (w385:refnum<k21>)
                    n278 = call <vilib>:"DAQmx Start Task.vi"("task/channels in"=w379, "error in"=w378) -> ("error out"=w380:errorcluster)  [unwired: 12 in, 1 out]
                    n279 = call <vilib>:"DAQmx Start Task.vi"("task/channels in"=w383, "error in"=w380) -> ("error out"=w384:errorcluster)  [unwired: 12 in, 1 out]
                    n280 = call <vilib>:"DAQmx Start Task.vi"("task/channels in"=w385, "error in"=w384) -> ()  [unwired: 12 in, 2 out]
                  }
                  frame #1 {
                    n281 = local read "motor panel"() -> (w394:T2)
                    n282 = Unbundle By Name(w394) -> ("Y destination"=w392:dbl)
                    n283 = local read "XPS Ref"() -> (w393:refnum<k24>)
                    n284 = local read "Y end"() -> (w390:dbl)
                    n285 = local read "speed"() -> (w389:dbl)
                    n286 = call "stage distance mode.vi"("Pos"=w392, "XPS Reference IN"=w393) -> ("LabVIEW error OUT"=w387:errorcluster, "Enable error"=w386:i32, "XPS Reference OUT"=w388:refnum<k24>)  [unwired: 6 in]
                    n287 = local write "Enable error"(w386) -> ()
                    n288 = call "stage control.vi"("Combo Box"="Y", "error in"=w387, "speed"=w389, "target"=w390, "XPS Ref in"=w388) -> ()  [unwired: 5 in, 2 out]
                  }
                }
              }
            }
          }
          frame "task imaging" {
            n289 = stacked-sequence {
              frame #0 {
                n290 = global read "params.vi" "NI tasks"() -> (w398:T4)
                n291 = Unbundle By Name(w398) -> ("frame trigger"=w400:refnum<k21>, "do"=w396:refnum<k21>, "digital galvo clock"=w399:refnum<k21>)
                n292 = call <vilib>:"DAQmx Start Task.vi"("task/channels in"=w399) -> ("error out"=w395:errorcluster)  [unwired: 13 in, 1 out]
                n293 = local read "main trigger"() -> (w402:refnum<k21>)
                n294 = call <vilib>:"DAQmx Start Task.vi"("task/channels in"=w396, "error in"=w395) -> ("error out"=w397:errorcluster)  [unwired: 12 in, 1 out]
                n295 = call <vilib>:"DAQmx Start Task.vi"("task/channels in"=w400, "error in"=w397) -> ("error out"=w401:errorcluster)  [unwired: 12 in, 1 out]
                n296 = call <vilib>:"DAQmx Start Task.vi"("task/channels in"=w402, "error in"=w401) -> ()  [unwired: 12 in, 2 out]
              }
              frame #1 {
                n297 = local read "task status"() -> (w417:T11)
                n298 = Unbundle By Name(w417) -> ("zn"=w415:u16, "xn"=w414:u16)
                n299 = local read "stage plan"() -> (w416:T1[][])
                n300 = Decrement(x=w415) -> (x-1=w412:u16)
                n301 = Decrement(x=w414) -> (x-1=w411:u16)
                n302 = Index Array(array=w416, index (row)=w412, index (col)=w411) -> (element=w413:T1)
                n303 = Unbundle By Name(w413) -> ("stage y start"=w405:dbl, "stage y end"=w408:dbl, "stage y speed"=w409:dbl)
                n304 = local read "XPS Ref"() -> (w406:refnum<k24>)
                n305 = call "stage distance mode.vi"("Pos"=w405, "XPS Reference IN"=w406) -> ("LabVIEW error OUT"=w404:errorcluster, "Enable error"=→"Enable error":i32, "XPS Reference OUT"=w407:refnum<k24>)  [unwired: 6 in]
                n306 = call "stage control.vi"("Combo Box"="Y", "error in"=w404, "speed"=w409, "target"=w408, "XPS Ref in"=w407) -> ()  [unwired: 5 in, 2 out]
              }
            }
          }
        }
        n307 = local write "acquisition finished"(FALSE ("acquisition finished")) -> ()
        n308 = Send Notification(notification="start acquisition", notifier=w369, error in (no error)=w371) -> (notifier out=w373:refnum<notifier>, error out=w367:errorcluster)
      }
      frame "during acquisition" {
        n309 = local write "current state"(w421) -> ()
      }
      frame "display" {
        n310 = local read "current frame index"() -> (w423:u16)
        n311 = Greater Than 0?(x=w423) -> (x > 0?=w422:bool)
        n312 = case shown="True" w422 {
          frame False {
          }
          frame True {
            # "rotate image adapt \nto user vision"
            n313 = local read "PXI channel"() -> (w435:T8)
            n314 = Unbundle By Name(w435) -> ("# of Channels"=w429:u8, "PMT2 # of Channels"=w428:u8)
            n315 = Add(x=w429, y=w428) -> (x+y=w427:u8)
            n316 = local read "PMT channel"() -> (w434:u8)
            n317 = Decrement(x=w427) -> (x-1=w432:u8)
            n318 = Less?(x=w434, y=w432) -> (x < y?=w433:bool)
            n319 = local read "images"() -> (w436:i16[][][])
            n320 = Select(t=w434, s=w433, f=w432) -> (s? t:f=w431:u8)
            n321 = local read "image"() -> (w437:T12)
            n322 = Index Array(array=w436, index (dim 0)=w431) -> (element=w430:i16[][])  [unwired: 2 in]
            n323 = call "IMAQ ArrayToImage"("Image Pixels (U16)"=w430, "Image"=w437) -> ("Image Out"=w438:T12)  [unwired: 8 in, 1 out]
            n324 = local write "image"(w438) -> ()
          }
        }
      }
      frame "finish acquisition" {
        n325 = local write "current state"(w444) -> ()
        n326 = stacked-sequence {
          tunnel: [w445 _] -> w443
          frame #0 {
            n327 = local read "imaging mode"() -> (w447:T5)
            n328 = local read "basic params"() -> (w446:T6)
            n329 = case shown="\"task imaging\"" w447 {
              tunnel: w446 -> [w449 _]
              tunnel: ["start acquisition" w463] -> w445
              frame "preview imaging", Default {
                n330 = Unbundle By Name(w449) -> ("stage scan?"=w450:bool)
                n331 = case shown="True" w450 {
                  frame False {
                    n332 = Wait (ms)(milliseconds to wait=u32 100) -> ()  [unwired: 1 out]
                  }
                  frame True {
                    n333 = local read "motor panel"() -> (w462:T2)
                    n334 = Unbundle By Name(w462) -> ("Y destination"=w455:dbl)
                    n335 = local read "XPS Ref"() -> (w456:refnum<k24>)
                    n336 = call "stage control.vi"("Combo Box"="Y", "speed"=10.0, "target"=w455, "XPS Ref in"=w456) -> ("error out"=w458:errorcluster, "XPS ref out"=w459:refnum<k24>)  [unwired: 6 in]
                    n337 = call "LWXPS_PositionerPositionCompareDisable.vi"("LabVIEW error IN"=w458, "Positioner Name"="Group2.Pos", "CommandInterfaceXPS.XPS"=w459) -> ()  [unwired: 3 in, 4 out]
                    n338 = local read "t"() -> (w454:dbl)
                    n339 = Add(x=w454, y=u32 1000 ("milliseconds to wait")) -> (x+y=w452:dbl)
                    n340 = Wait (ms)(milliseconds to wait=w452) -> ()  [unwired: 1 out]
                  }
                }
              }
              frame "task imaging" {
                n341 = local read "task status"() -> (w465:T11)
                n342 = local read "task plan"() -> (w468:T10)
                n343 = local read "stage plan"() -> (w464:T1[][])
                n344 = Unbundle By Name(w465) -> ("scan n"=w466:u16)
                n345 = Unbundle By Name(w468) -> ("end scan #"=w467:u16)
                n346 = Equal?(x=w466, y=w467) -> (x = y?=w469:bool)
                n347 = case shown="False" w469 {
                  tunnel: w466 -> [w503 _]
                  tunnel: w465 -> [w506 _]
                  tunnel: w464 -> [w499 _]
                  tunnel: ["start acquisition" "finish task"] -> w463
                  frame False {
                    n348 = Array Size(array=w499) -> (size(s)=w502:i32[])
                    n349 = Index Array(array=w502, index=1) -> (element=w500:i32)
                    n350 = Increment(x=w503) -> (x+1=w504:u16)
                    n351 = Quotient & Remainder(x=w503, y=w500) -> (x-y*floor(x/y)=w493:i32, floor(x/y)=w494:i32)
                    n352 = Increment(x=w494) -> (x+1=w496:i32)
                    n353 = Increment(x=w493) -> (x+1=w495:i32)
                    n354 = Index Array(array=w499, index (row)=w494, index (col)=w493) -> (element=w498:T1)
                    n355 = Unbundle By Name(w498) -> ("stage x"=w471:dbl, "stage y start"=w470:dbl, "stage y end"=w491:dbl, "stage z"=w480:dbl)
                    n356 = Bundle By Name(cluster=w506, "scan n"=w504, "zn"=w496, "xn"=w495) -> (w505:T11)
                    n357 = local read "XPS Ref"() -> (w479:refnum<k24>)
                    n358 = Subtract(x=w470, y=w491) -> (x-y=w484:dbl)
                    n359 = local write "task status"(w505) -> ()
                    n360 = Absolute Value(x=w484) -> (abs(x)=w483:dbl)
                    n361 = call "stage control.vi"("Combo Box"="Y", "speed"=10.0, "target"=w470, "XPS Ref in"=w479) -> ("error out"=w477:errorcluster, "XPS ref out"=w478:refnum<k24>)  [unwired: 6 in]
                    n362 = Divide(x=w483, y=10.0) -> (x/y=w489:dbl)
                    n363 = call "stage control.vi"("Combo Box"="Z", "error in"=w477, "speed"=5.0, "target"=w480, "XPS Ref in"=w478) -> ("error out"=w475:errorcluster, "XPS ref out"=w472:refnum<k24>)  [unwired: 5 in]
                    n364 = Multiply(x=w489, y=1000.0) -> (x*y=w487:dbl)
                    n365 = Add(x=w487, y=2000.0) -> (x+y=w485:dbl)
                    n366 = call "stage control.vi"("Combo Box"="X", "error in"=w475, "speed"=10.0, "target"=w471, "XPS Ref in"=w472) -> ()  [unwired: 5 in, 2 out]
                    n367 = Wait (ms)(milliseconds to wait=w485) -> ()  [unwired: 1 out]
                  }
                  frame True {
                  }
                }
              }
            }
          }
          frame #1 {
            n368 = global read "params.vi" "NI tasks"() -> (w510:T4)
            n369 = Unbundle By Name(w510) -> ("do"=w509:refnum<k21>, "digital galvo clock"=w508:refnum<k21>)
            n370 = call <vilib>:"DAQmx Stop Task.vi"("task/channels in"=w509) -> ()  [unwired: 13 in, 2 out]
            n371 = call <vilib>:"DAQmx Stop Task.vi"("task/channels in"=w508) -> ()  [unwired: 13 in, 2 out]
          }
        }
        n372 = local read "current frame index"() -> (w440:u16)
        n373 = Increment(x=w440) -> (x+1=w439:u16)
        n374 = local write "current frame index"(w439) -> ()
      }
      frame "finish task" {
        w525 = T13."Enabled" ("Disabled")
        n375 = local write "current state"(w533) -> ()
        n376 = local read "imaging mode"() -> (w522:T5)
        n377 = local read "main trigger"() -> (w523:refnum<k21>)
        n378 = case shown="\"preview imaging\", Default" w522 {
          tunnel: [w538 w540] -> w519
          frame "preview imaging", Default {
            n379 = local read "motor panel"() -> (w539:T2)
            n380 = Unbundle By Name(w539) -> ("Y destination"=w538:dbl)
          }
          frame "task imaging" {
            n381 = local read "stage plan"() -> (w544:T1[][])
            n382 = Index Array(array=w544, index (row)=0, index (col)=0 ("disabled index (col)")) -> (element=w541:T1)
            n383 = Unbundle By Name(w541) -> ("stage y start"=w540:dbl)
          }
        }
        n384 = call <vilib>:"DAQmx Clear Task.vi"("task in"=w523) -> ("error out"=w511:errorcluster)  [unwired: 14 in]
        n385 = flat-sequence {
          tunnel: [w537] -> w512
          tunnel: w511 -> [w537]
          frame #0 {
            n386 = Wait (ms)(milliseconds to wait=u32 2000) -> ()  [unwired: 1 out]
          }
        }
        n387 = local read "XPS Ref"() -> (w515:refnum<k24>)
        n388 = call "LWXPS_PositionerPositionCompareDisable.vi"("LabVIEW error IN"=w512, "Positioner Name"="Group2.Pos", "CommandInterfaceXPS.XPS"=w515) -> ("LabVIEW error OUT"=w514:errorcluster, "CommandInterfaceXPS.XPS"=w513:refnum<k24>)  [unwired: 3 in, 2 out]
        n389 = call "stage control.vi"("Combo Box"="Y", "error in"=w514, "speed"=10.0, "target"=w519, "XPS Ref in"=w513) -> ()  [unwired: 5 in, 2 out]
        n390 = local write "Acquire"(FALSE ("Acquire")) -> ()
        n391 = property on="imaging mode" class="CmbBox (strict)"("DisabledEnum"=w525) -> ()  [unwired: 2 in, 2 out]
        n392 = property on="basic params" class="Clust (strict)"("DisabledEnum"=w525) -> ()  [unwired: 2 in, 2 out]
        n393 = property on="PXI channel" class="Clust (strict)"("DisabledEnum"=w525) -> ()  [unwired: 2 in, 2 out]
        n394 = property on="Calc Waveform" class="Bool (strict)"("DisabledEnum"=w525) -> ()  [unwired: 2 in, 2 out]
        n395 = property on="Stop" class="Bool (strict)"("DisabledEnum"=w525) -> ()  [unwired: 2 in, 2 out]
        n396 = property on="motor panel" class="Clust (strict)"("DisabledEnum"=w525) -> ()  [unwired: 2 in, 2 out]
        n397 = property on="advanced params" class="Clust (strict)"("DisabledEnum"=w525) -> ()  [unwired: 2 in, 2 out]
        n398 = property on="task plan" class="Clust (strict)"("DisabledEnum"=w525) -> ()  [unwired: 2 in, 2 out]
        n399 = global read "params.vi" "NI tasks"() -> (w526:T4)
        n400 = Unbundle By Name(w526) -> ("frame trigger"=w530:refnum<k21>, "PMT in"=w529:refnum<k15>, "do"=w528:refnum<k21>, "digital galvo clock"=w527:refnum<k21>, "PMT2 in"=w524:refnum<k15>)
        n401 = call <vilib>:"DAQmx Clear Task.vi"("task in"=w530) -> ()  [unwired: 14 in, 1 out]
        n402 = call <instrlib>:"niScope Close.vi"("instrument handle"=w529) -> ()  [unwired: 14 in, 1 out]
        n403 = call <vilib>:"DAQmx Clear Task.vi"("task in"=w528) -> ("error out"=w521:errorcluster)  [unwired: 14 in]
        n404 = call <vilib>:"DAQmx Clear Task.vi"("task in"=w527, "error in"=w521) -> ("error out"=w520:errorcluster)  [unwired: 13 in]
        n405 = call <instrlib>:"niScope Close.vi"("instrument handle"=w524) -> ()  [unwired: 14 in, 1 out]
        n406 = call "digital galvo position ver2.vi"("error in"=w520) -> ()  [unwired: 10 in, 1 out]
      }
      frame "exit", Default {
        # "save to last configuration"
        n407 = local write "current state"(w552) -> ()
        n408 = Send Notification(notification="stop", notifier=w550, error in (no error)=w548) -> (notifier out=w549:refnum<notifier>, error out=w547:errorcluster)
        n409 = call <vilib>:"Application Directory.vi"() -> ("Application Directory"=w546:path)
        n410 = call "save configuration.vi"("filename"="last configuration.ini" ("name or relative path"), "path"=w546) -> ()  [unwired: 9 in, 1 out]
      }
    }
  }
  n411 = while {
    tunnel: w3 -> [w555]
    tunnel: w10 -> [w556]
    stop <- w557 stop-if-true
    n412 = Wait on Notification(notifier=w555) -> (notification=w558:string)  [unwired: 1 in, 5 out]
    n413 = case shown="\"start acquisition\"" w558 {
      tunnel: [_ _ TRUE] -> w557
      tunnel: w556 -> [_ w560 _]
      tunnel: w555 -> [_ w559 _]
      frame "False", Default {
      }
      frame "start acquisition" {
        n414 = stacked-sequence {
          tunnel: w560 -> [_ w583 _ _]
          tunnel: w559 -> [_ w582 _ _]
          frame #0 {
            n415 = global read "params.vi" "NI tasks"() -> (w564:T4)
            n416 = Unbundle By Name(w564) -> ("PMT in"=w563:refnum<k15>, "PMT2 in"=w561:refnum<k15>)
            n417 = call <instrlib>:"niScope Initiate Acquisition.vi"("instrument handle"=w563) -> ("error out"=w562:errorcluster)  [unwired: 13 in, 1 out]
            n418 = call <instrlib>:"niScope Initiate Acquisition.vi"("instrument handle"=w561, "error in"=w562) -> ()  [unwired: 12 in, 2 out]
          }
          frame #1 {
            n419 = local read "basic params"() -> (w576:T6)
            n420 = local read "advanced params"() -> (w575:T7)
            n421 = local read "PXI channel"() -> (w574:T8)
            n422 = global read "params.vi" "NI tasks"() -> (w577:T4)
            n423 = Unbundle By Name(w576) -> ("Y pixel #"=w585:u32)
            n424 = Unbundle By Name(w574) -> ("# of Channels"=w580:u8, "PMT2 # of Channels"=w566:u8)
            n425 = Unbundle By Name(w575) -> ("fetch # per frame"=w579:u16)
            n426 = Divide(x=w585, y=2) -> (x/y=w584:dbl)
            n427 = Unbundle By Name(w577) -> ("PMT in"=w586:refnum<k15>)
            n428 = Unbundle By Name(w577) -> ("PMT2 in"=w572:refnum<k15>)
            n429 = Divide(x=w584, y=w579) -> (x/y=w578:dbl)
            n430 = call "convert channel number into DAQ channel string.vi"("Numeric"=w580) -> ("String"=w581:string)  [unwired: 10 in]
            n431 = call "convert channel number into DAQ channel string.vi"("Numeric"=w566) -> ("String"=w571:string)  [unwired: 10 in]
            n432 = while {
              tunnel: w578 -> [w620]
              tunnel: w579 -> [w615]
              tunnel: w581 -> [w619]
              tunnel: w586 -> [w618]
              tunnel: [w610] -> w567 mode=concatenating
              tunnel: [w607] -> w565 mode=concatenating
              tunnel: w572 -> [w604]
              tunnel: w571 -> [w603]
              i -> [w617]
              stop <- w621 stop-if-true
              n433 = Multiply(x=w620, y=w617) -> (x*y=w606:dbl)
              n434 = Increment(x=w617) -> (x+1=w616:i32)
              n435 = property class="niScope"(reference=w618, "Fetch Record Number"=w606) -> (reference out=w613:refnum<k15>, error out=w612:errorcluster)  [unwired: 1 in]
              n436 = Equal?(x=w616, y=w615) -> (x = y?=w614:bool)
              n437 = local read "Acquire"() -> (w623:bool)
              n438 = Not(x=w623) -> (.not. x?=w622:bool)
              n439 = Compound Arithmetic op=OR(w622, w614) -> (w621:bool)
              n440 = call-poly <instrlib>:"niScope Fetch (poly).vi"("timeout"=10.0, "error in"=w612, "channels"=w619, "instrument handle"=w613) -> ("error out"=w605:errorcluster, "wfm"=w610:i16[][])  [unwired: 4 in, 2 out]
              n441 = property class="niScope"(reference=w604, error in=w605, "Fetch Record Number"=w606) -> (reference out=w609:refnum<k15>, error out=w608:errorcluster)
              n442 = call-poly <instrlib>:"niScope Fetch (poly).vi"("error in"=w608, "channels"=w603, "instrument handle"=w609) -> ("wfm"=w607:i16[][])  [unwired: 5 in, 3 out]
            }
            n443 = local read "imaging mode"() -> (w573:T5)
            n444 = Insert Into Array(array=w567, new element=w565) -> (w570:i16[][])  [unwired: 2 in]
            n445 = case shown="\"False\", Default" w573 {
              tunnel: w583 -> [_ w602]
              tunnel: w582 -> [_ w601]
              tunnel: w576 -> [w593 _]
              tunnel: w575 -> [w592 _]
              tunnel: w574 -> [w591 _]
              tunnel: w570 -> [_ w598]
              tunnel: w567 -> [w597 _]
              tunnel: w565 -> [w596 _]
              frame "False", Default {
                n446 = global read "params.vi" "x flyback pixel"() -> (w594:u16)
                n447 = call "reconstruct single image for display.vi"("bidirection?"="bi? for display", "x fly back pixel"=w594, "PXI channel"=w591, "advanced params"=w592, "basic params"=w593, "raw data"=w597) -> ("images"=w590:i16[][][])  [unwired: 5 in]
                n448 = call "reconstruct single image for saving channel 2.vi"("bidirection?"="bi? for display", "x fly back pixel"=w594, "PXI channel"=w591, "advanced params"=w592, "basic params"=w593, "raw data"=w596) -> ("images"=w589:i16[][][])  [unwired: 5 in]
                n449 = Insert Into Array(array=w590, new element=w589) -> (→"images":i16[][][])  [unwired: 3 in]
              }
              frame "task imaging" {
                n450 = Enqueue Element(queue=w602, element=w598) -> (error out=w599:errorcluster)  [unwired: 2 in, 2 out]
                n451 = Send Notification(notification="new data in quene", notifier=w601, error in (no error)=w599) -> ()  [unwired: 2 out]
              }
            }
            n452 = Array Size(array=w567) -> (size(s)=→"PMT array size":i32[])
            n453 = Array Size(array=w565) -> (size(s)=→"PMT2 array size":i32[])
          }
          frame #2 {
            n454 = global read "params.vi" "NI tasks"() -> (w626:T4)
            n455 = Unbundle By Name(w626) -> ("frame trigger"=w628:refnum<k21>, "PMT in"=w627:refnum<k15>, "PMT2 in"=w625:refnum<k15>)
            n456 = local read "main trigger"() -> (w624:refnum<k21>)
            n457 = call <vilib>:"DAQmx Stop Task.vi"("task/channels in"=w624) -> ()  [unwired: 13 in, 2 out]
            n458 = call <vilib>:"DAQmx Stop Task.vi"("task/channels in"=w628) -> ()  [unwired: 13 in, 2 out]
            n459 = call <instrlib>:"niScope Abort.vi"("instrument handle"=w627) -> ()  [unwired: 13 in, 2 out]
            n460 = call <instrlib>:"niScope Abort.vi"("instrument handle"=w625) -> ()  [unwired: 13 in, 2 out]
          }
          frame #3 {
            n461 = local write "acquisition finished"(TRUE ("acquisition finished")) -> ()
          }
        }
      }
      frame "stop" {
      }
    }
  }
  n462 = while {
    tunnel: w10 -> [w634]
    tunnel: w3 -> [w633]
    stop <- w631 stop-if-true
    n463 = Wait on Notification(notifier=w633) -> (notification=w632:string)  [unwired: 3 in, 3 out]
    n464 = case shown="\"new data in quene\"" w632 {
      tunnel: w634 -> [_ w635 w697]
      tunnel: [_ _ TRUE] -> w631
      frame "False", Default {
      }
      frame "new data in quene" {
        n465 = while {
          tunnel: w635 -> [w647]
          stop <- w643 stop-if-true
          n466 = local read "basic params"() -> (w641:T6)
          n467 = local read "advanced params"() -> (w640:T7)
          n468 = local read "PXI channel"() -> (w639:T8)
          n469 = local read "task status"() -> (w636:T11)
          n470 = local read "PMT array size"() -> (w642:i32[])
          n471 = local read "PMT2 array size"() -> (w637:i32[])
          n472 = global read "params.vi" "x flyback pixel"() -> (w638:u16)
          n473 = Get Queue Status(queue=w647) -> (queue out=w646:refnum<queue>, # elements in queue=w645:i32)  [unwired: 2 in, 6 out]
          n474 = Not Equal To 0?(x=w645) -> (x != 0?=w644:bool)
          n475 = case shown="True" w644 {
            tunnel: w646 -> [_ w686]
            tunnel: w640 -> [_ w676]
            tunnel: w636 -> [_ w685]
            tunnel: w641 -> [_ w673]
            tunnel: w638 -> [_ w677]
            tunnel: [TRUE _] -> w643
            tunnel: w639 -> [_ w675]
            tunnel: w642 -> [_ w665]
            tunnel: w641 -> [_ w655]
            tunnel: w640 -> [_ w654]
            tunnel: w639 -> [_ w653]
            tunnel: w638 -> [_ w656]
            tunnel: w637 -> [_ w662]
            frame False {
            }
            frame True {
              w670 = 0 ("index")
              # "rawdata bidirection"
              n476 = Dequeue Element(queue=w686) -> (element=w666:i16[][])  [unwired: 2 in, 3 out]
              n477 = Unbundle By Name(w685) -> ("write"=w674:u16)
              n478 = Index Array(array=w662, index=0) -> (element=w661:i32)
              n479 = Index Array(array=w665, index=0) -> (element=w671:i32)
              n480 = Index Array(array=w665, index=0) -> (element=w664:i32)
              n481 = Array Subset(array=w666, index (row)=w670, length (row)=w671, index (col)=w670) -> (w669:i16[][])  [unwired: 1 in]
              n482 = Array Subset(array=w666, index (row)=w664, length (row)=w661, index (col)=0 ("index")) -> (w657:i16[][])  [unwired: 1 in]
              n483 = Increment(x=w674) -> (x+1=w658:u16)
              n484 = call "reconstruct single image for display.vi"("bidirection?"="bi? for save", "x fly back pixel"=w677, "PXI channel"=w675, "advanced params"=w676, "basic params"=w673, "raw data"=w669) -> ("images"=w651:i16[][][])  [unwired: 5 in]
              n485 = call "reconstruct single image for saving channel 2.vi"("bidirection?"="bi? for save", "x fly back pixel"=w656, "PXI channel"=w653, "advanced params"=w654, "basic params"=w655, "raw data"=w657) -> ("images"=w650:i16[][][])  [unwired: 5 in]
              n486 = local read "file path"() -> (w683:path)
              n487 = Insert Into Array(array=w651, new element=w650) -> (w649:i16[][][])  [unwired: 3 in]
              n488 = for {
                tunnel: [w695] -> w678 mode=indexing
                tunnel: w649 -> [w689] mode=indexing
                i -> [w691]
                w694 = T14 7 items=["Grayscale (U8)", "Grayscale (I16)", "Grayscale (SGL)", "Complex (CSG)", "RGB (U32)", "HSL (U32)", "RGB (U64)", "Grayscale (U16)"] ("Image Type")
                n489 = Number To Decimal String(number=w691, width (-)=i16 3) -> (decimal integer string=w692:string)
                n490 = call "IMAQ Create"("Image Name"=w692, "Image Type"=w694) -> ("New Image"=w690:T12)  [unwired: 3 in, 1 out]
                n491 = call "IMAQ ArrayToImage"("Image Pixels (U16)"=w689, "Image"=w690) -> ("Image Out"=w695:T12)  [unwired: 8 in, 1 out]
              }
              n492 = Bundle By Name(cluster=w685, "write"=w658) -> (w679:T11)
              n493 = Strip Path(path=w683) -> (stripped path=w660:path, name=w659:string)
              n494 = local write "images"(w649) -> ()
              n495 = local write "task status"(w679) -> ()
              n496 = Format Value(string ("")=w659, format string="_%05u.tif", value (0)=w658) -> (output string=w681:string)
              n497 = Build Path(base path=w660, name or relative path=w681) -> (appended path=w682:path)
              n498 = call "Save multiple images to new tiff stack.vi"("Array of Images (U8, U16, I16)"=w678, "Path"=w682) -> ("error out"=w680:errorcluster)  [unwired: 9 in]
              n499 = for {
                tunnel: w680 -> [w688]
                tunnel: w678 -> [w687] mode=indexing
                n500 = call "IMAQ Dispose"("Image"=w687, "error in (no error)"=w688) -> ()  [unwired: 4 in, 1 out]
              }
            }
          }
        }
      }
      frame "stop" {
        n501 = Release Queue(queue=w697) -> ()  [unwired: 2 in, 3 out]
      }
    }
  }
  n502 = flat-sequence {
    tunnel: w9 -> [w700]
    tunnel: [w700] -> w8
    tunnel: w5 -> [w699]
    tunnel: [w699] -> w7
    frame #0 {
      # "wait for slave loop"
      n503 = Wait (ms)(milliseconds to wait=u32 500) -> ()  [unwired: 1 out]
    }
  }
  n504 = Release Notifier(notifier=w8, error in (no error)=w7) -> ()  [unwired: 4 out]
